vi "translate_digital_inputs.vi"(2 "di_value (in)":u32) -> (16 "dig_in_value (out)":u32, 17 "dig_in_items (out)":T1[](array[typedef]))   [LabVIEW 2012]
doc: "Translates the digital input values FROM the numeric value returned via the API call.\n\nProduced By:\n\nChristopher Lemieux\nKod Integrations, LLC\n4835 Marianne Drive\nMount Airy, MD 21771\nhttp://www.kodintegrations.com\nemail: clemieux@kodintegrations.com\nphone: (240) 687-1288"
uses:
  controls/digital_input_item_group.ctl
  controls/digital_input_items.ctl
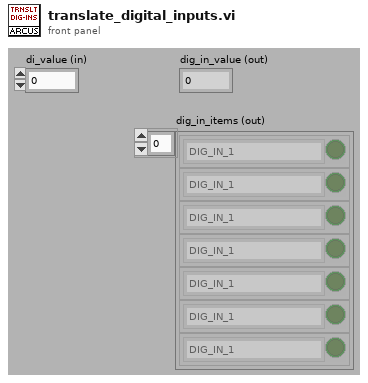
[diagram p1: front panel]
types:
  T1 = typedef "digital_input_item_group.ctl" = cluster{"item":T2, "status":bool}
  T2 = typedef "digital_input_items.ctl" = enum16{"DIG_IN_1", "DIG_IN_2", "NEG_LIMIT", "HOME", "POS_LIMIT"}
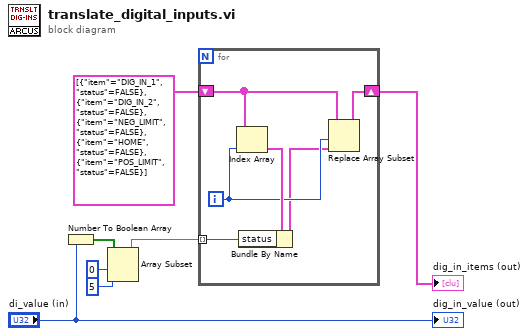
[diagram p0: block diagram]
diagram:
  n1 = Number To Boolean Array(number="di_value (in)") -> (Boolean array=w4:bool[])
  n2 = Array Subset(array=w4, index=0, length=5) -> (w1:bool[])
  n3 = for {
    shift-right: [w8] -> w7
    shift-left: T1[] [{"item"=enum."DIG_IN_1", "status"=FALSE}, {"item"=enum."DIG_IN_2", "status"=FALSE}, {"item"=enum."NEG_LIMIT", "status"=FALSE}, {"item"=enum."HOME", "status"=FALSE}, {"item"=enum."POS_LIMIT", "status"=FALSE}] ("polarity_items (in)") -> [w11]
    tunnel: w1 -> [w12] mode=indexing
    i -> [w10]
    n4 = Index Array(array=w11, index=w10) -> (element=w13:T1)
    n5 = Bundle By Name(cluster=w13, "status"=w12) -> (w9:T1)
    n6 = Replace Array Subset(array=w11, new element=w9, index=w10) -> (w8:T1[])
  }
  "dig_in_items (out)" <- w7
  "dig_in_value (out)" <- "di_value (in)"
